vi "ProcessBufferUpdates.vi"(11 "MockFAILCSettings":T1={"ModbusRxDataFIFO"="ModbusSubnetARxDataFIFO", "ModbusTxDataFIFO"="ModbusSubnetATxDataFIFO", "BufferUpdateFIFO"="MockFAILC1Command", "Code17Memory"="MockFAILC1Code17", "Code18Memory"="MockFAILC1Code18", "Code65Memory"="MockFAILC1Code65", "Code72Memory"="MockFAILC1Code72", "Code74Memory"="MockFAILC1Code74", "Code75Memory"="MockFAILC1Code75", "Code76Memory"="MockFAILC1Code76", "Code80Memory"="MockFAILC1Code80", "Code110Memory"="MockFAILC1Code110", "Code120Memory"="MockFAILC1Code120", "Code121Memory"="MockFAILC1Code121", "CRCDataFIFO"="MockFAILC1CRCDataFIFO", "CRCCalculateFIFO"="MockFAILC1CRCCalculateFIFO", "CRCFIFO"="MockFAILC1CRCFIFO"}) -> ()   [LabVIEW 2016, in "FPGAMockFAILC.lvlib"]
uses:
  FPGAMockFAILC.lvlib
  DataTypes/MockFAILCSettings.ctl
  FPGAMockHPILC/DataTypes/MockHPBufferUpdateLoopData.ctl
  FPGAMockHPILC/DataTypes/MockHPBufferUpdateStates.ctl
  <vilib>/Platform/TimedLoop/XDataNode/timing_clust.ctl
  <vilib>/Platform/TimedLoop/XDataNode/nitl_modes.ctl
  <vilib>/Platform/TimedLoop/XDataNode/wakeup.ctl
  <vilib>/rvi/Emulation/niFpgaSctlEmulationGetInTimedLoop.vi
  <vilib>/rvi/Emulation/niFpgaEmulationReportErrorSimple.vi
  <vilib>/rvi/Emulation/niFpgaGetClockAttributes.vi
  <vilib>/rvi/Emulation/niFpgaCriticalErrorInLSC.vi
  <vilib>/rvi/DataTransferAndStorage/Container/Common/niFpgaContainerExecOnDevCompGetState.vi
  <vilib>/rvi/Emulation/niFpgaEmulationIsFPGAContextNoSignature.vi
  <vilib>/rvi/errors/niFpgaSetErrorForExecOnDevCompSimple.vi
  <vilib>/rvi/eio/common/nirviEmuReportErrorAndStop.vi
  <vilib>/rvi/DataTransferAndStorage/Container/Common/niFpgaContainerGetUniqueNameForEmu.vi
  <vilib>/rvi/FIFO/Fifo_Resource/nirvififoEmulationSetSize.vi
  <vilib>/rvi/FIFO/Fifo_Resource/nirviFifoEmulationQueueMgr.vi
  <instcachedir>/0/nirviFifoEmulationQueueMgr_E5CAEC123FF24DC58D834DCA3CDAA9B5.lvgen/nirviFifoEmulationQueueMgr_E5CAEC123FF24DC58D834DCA3CDAA9B5_009.vi
  <vilib>/rvi/FIFO/Fifo_Resource/nirvififoEmulationDetermineInputValidOut.vi
  <vilib>/rvi/FIFO/Fifo_Resource/nirvififoEmulationCreateLock.vi
  <vilib>/rvi/Emulation/niFpgaProcessEmulError.vi
  <vilib>/rvi/FIFO/Fifo_Resource/nirvififoEmulationObtainLock.vi
  <vilib>/rvi/FIFO/Fifo_Resource/nirvififoEmulationReleaseLock.vi
  <vilib>/rvi/occurrence/nirviWaitOnOccurrenceBase.vi
  <vilib>/rvi/errors/nirviReportUnexpectedCaseInternalError.vi
  <vilib>/rvi/errors/nirviReportUnexpectedCaseInternalError (U32).vi
  <vilib>/Utility/error.llb/Clear Errors.vi
  <vilib>/rvi/interface/RandomDataEmulation/niFpgaRandomDataHandleErrors.vi
  <vilib>/rvi/Memory/Memory_Emulation/niFpgaMemoryEmulationCacheClearOnFirstRun.vi
  <vilib>/rvi/Memory/Memory_Emulation/nirvimemoryEmulationManagerCache_MakeExclusive.vi
  <vilib>/rvi/Memory/Memory_Emulation/niFpgaMemoryEmulationValidateCache.vi
  <vilib>/rvi/Memory/Memory_Emulation/nirvimemoryEmulationManagerCache_InsertValue.vi
  <vilib>/rvi/Memory/Memory_Emulation/nirvimemoryEmulationManagerCache_ReleaseExclusive.vi
  <vilib>/rvi/Memory/Memory_Emulation/nirvimemoryEmulationManagerCache_GetValue.vi
  <vilib>/rvi/Memory/Memory_Emulation/nirvimemoryEmulationManagerCache_SetValue.vi
  <vilib>/rvi/Emulation/niFpgaSctlEmulationResourceMgr.vi
  <vilib>/Platform/TimedLoop/XDataNode/XDataNode.xnode
  <vilib>/rvi/DataTransferAndStorage/Container/XNode/niFpgaContainer.xnode
  <vilib>/rvi/FIFO/Fifo_Resource/niFpgaFifoEmulationRefIn.vi
  <vilib>/rvi/Memory/Memory_Emulation/niFpgaMemoryEmulationRefIn.vi
  <vilib>/Platform/TimedLoop/XDataNode/XDNodeRunTimeDep.lvlib
  FPGAMockHPILC/FPGAMockHPILC.lvlib
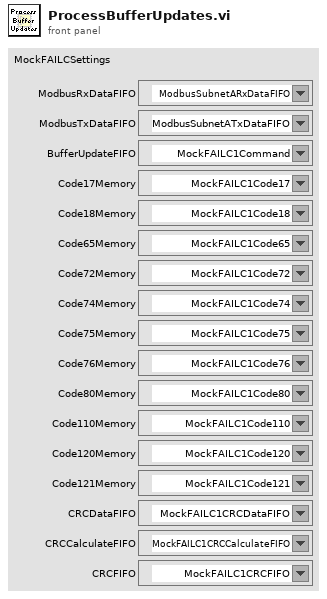
[diagram p1: front panel]
types:
  T1 = typedef "FPGAMockFAILC.lvlib/MockFAILCSettings.ctl" = cluster{"ModbusRxDataFIFO":refnum<k21>, "ModbusTxDataFIFO":refnum<k21>, "BufferUpdateFIFO":refnum<k21>, "Code17Memory":refnum<k21>, "Code18Memory":refnum<k21>, "Code65Memory":refnum<k21>, "Code72Memory":refnum<k21>, "Code74Memory":refnum<k21>, "Code75Memory":refnum<k21>, "Code76Memory":refnum<k21>, "Code80Memory":refnum<k21>, "Code110Memory":refnum<k21>, "Code120Memory":refnum<k21>, "Code121Memory":refnum<k21>, "CRCDataFIFO":refnum<k21>, "CRCCalculateFIFO":refnum<k21>, "CRCFIFO":refnum<k21>}
  T2 = typedef "FPGAMockHPILC.lvlib/MockHPBufferUpdateLoopData.ctl" = cluster{"BufferUpdateLoopStates":T3, "Address":u32, "Function":u8, "Length":u32, "Data":u8, "Index":u32}
  T3 = typedef "FPGAMockHPILC.lvlib/MockHPBufferUpdateStates.ctl" = enum16{"ReadAddress", "ReadFunction", "ReadLength", "ReadData", "WriteData"}
  T4 = typedef "XDNodeRunTimeDep.lvlib/timing_clust.ctl" = cluster{"Expected End [f-1]":u64, "Actual End [f-1]":u64, "Finished Late? [f-1]":bool, "Expected End [i-1]":u64, "Actual End [i-1]":u64, "Finished Late? [i-1]":bool, "Expected Start [i]":u64, "Actual Start [i]":u64, "Expected Start [f]":u64, "Actual Start [f]":u64, "Source Name":string, "Structure Name":string, "Period":i64, "Deadline":i64, "Offset":i64, "Start":i64, "Priority":i32, "Timeout":i32, "Mode":T5, "Wakeup Reason":T6, "Error":errorcluster, "Source Type":string, "Secondary Source Type":string, "Global End Time":u64, "Global Start Time":u64, "Frame Duration":u64, "Iteration Duration":u64, "Assigned CPU":i32, "I/O Scan Engine Mode":u32}
  T5 = typedef "XDNodeRunTimeDep.lvlib/nitl_modes.ctl" = enum32{"No Change", "Process missed periods, maintain original phase", "Discard missed periods, maintain original phase", "Process missed periods, ignore original phase", "Discard missed periods, ignore original phase"}
  T6 = typedef "XDNodeRunTimeDep.lvlib/wakeup.ctl" = enum32{"Normal", "Aborted", "Asynchronous wakeup", "Timing source error", "Timed loop error", "Timeout"}
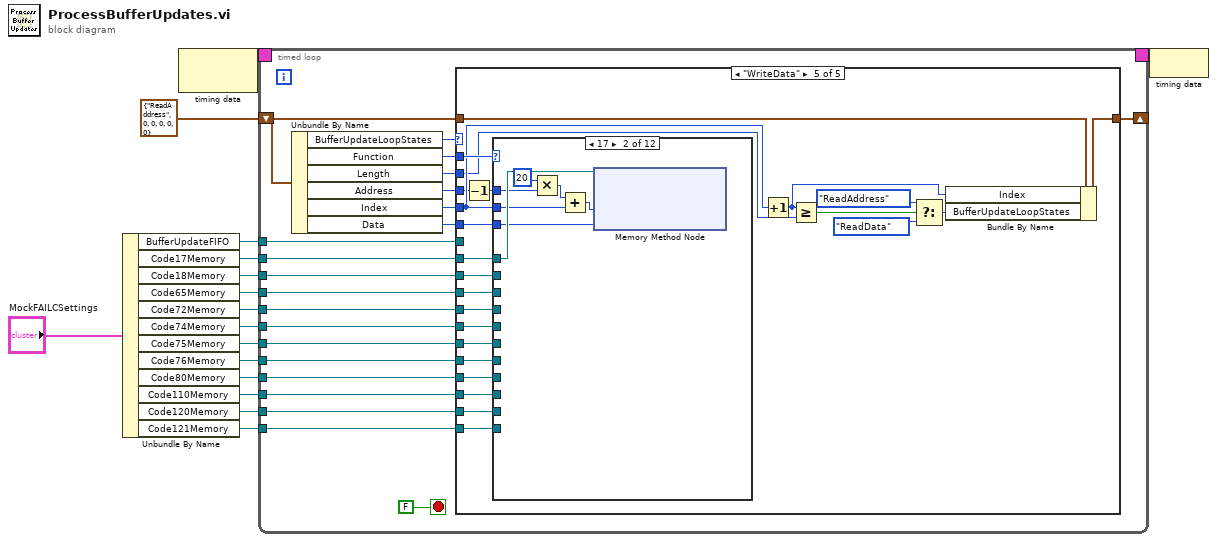
[diagram p0: block diagram]
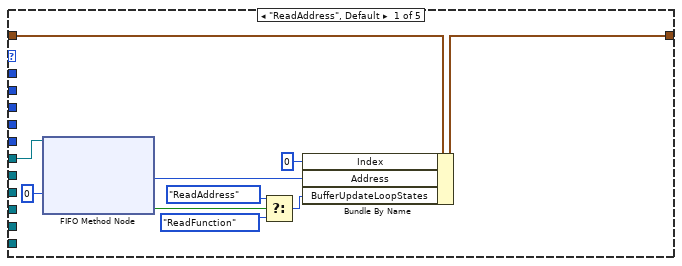
[diagram p2: hidden frame]
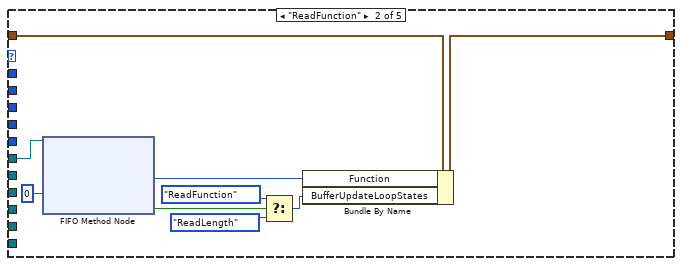
[diagram p3: hidden frame]
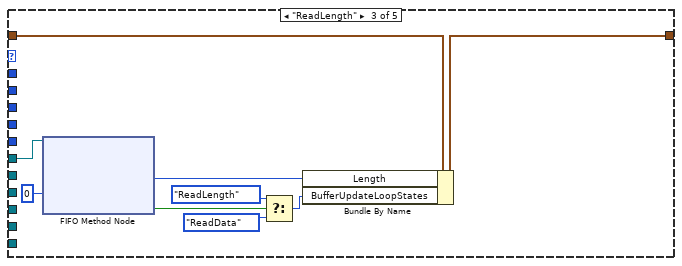
[diagram p4: hidden frame]
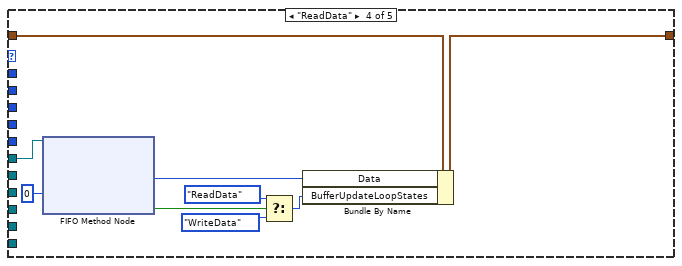
[diagram p5: hidden frame]
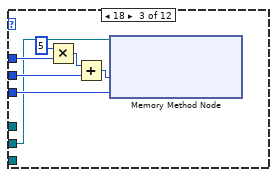
[diagram p7: hidden frame]
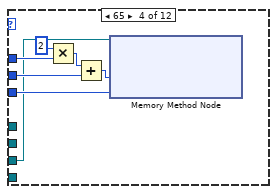
[diagram p8: hidden frame]
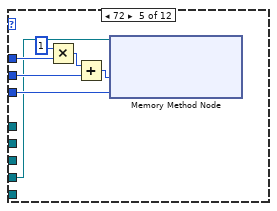
[diagram p9: hidden frame]
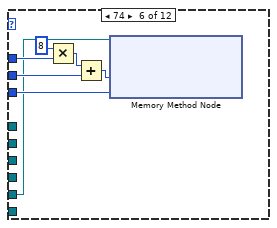
[diagram p10: hidden frame]
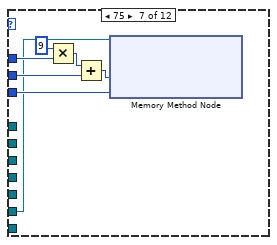
[diagram p11: hidden frame]
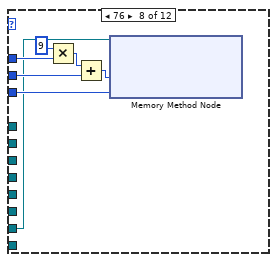
[diagram p12: hidden frame]
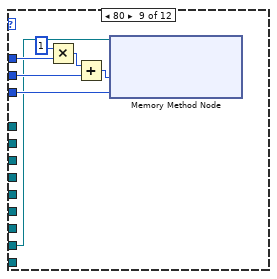
[diagram p13: hidden frame]
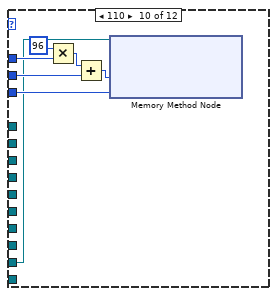
[diagram p14: hidden frame]
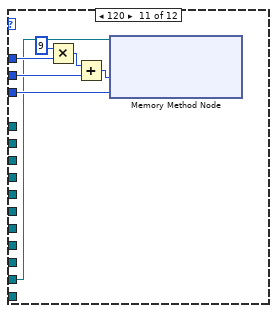
[diagram p15: hidden frame]
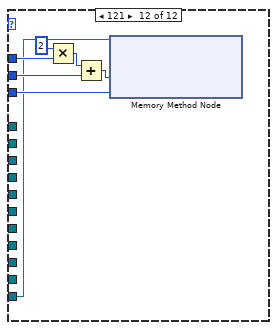
[diagram p16: hidden frame]
diagram:
  n1 = Unbundle By Name("MockFAILCSettings") -> ("BufferUpdateFIFO"=w13:refnum<k21>, "Code17Memory"=w12:refnum<k21>, "Code18Memory"=w11:refnum<k21>, "Code65Memory"=w10:refnum<k21>, "Code72Memory"=w9:refnum<k21>, "Code74Memory"=w8:refnum<k21>, "Code75Memory"=w7:refnum<k21>, "Code76Memory"=w6:refnum<k21>, "Code80Memory"=w5:refnum<k21>, "Code110Memory"=w3:refnum<k21>, "Code120Memory"=w2:refnum<k21>, "Code121Memory"=w1:refnum<k21>)
  n2 = node-c288() -> (w16:T4)  [unwired: 1 in]
  n3 = timed-loop {
    timing: w16 -> [_]
    timing-out: [_] -> w15
    tunnel: w13 -> [w36]
    tunnel: w12 -> [w28]
    tunnel: w11 -> [w27]
    tunnel: w10 -> [w26]
    tunnel: w9 -> [w25]
    tunnel: w8 -> [w24]
    tunnel: w7 -> [w23]
    tunnel: w6 -> [w22]
    tunnel: w5 -> [w21]
    shift-right: [w30] -> _
    shift-left: T2 {"BufferUpdateLoopStates"=enum."ReadAddress", "Address"=0, "Function"=0, "Length"=0, "Data"=0, "Index"=0} ("MockHPBufferUpdateLoopData") -> [w35]
    tunnel: w3 -> [w19]
    tunnel: w2 -> [w18]
    tunnel: w1 -> [w17]
    stop <- FALSE stop-if-true
    n4 = Unbundle By Name(w35) -> ("BufferUpdateLoopStates"=w37:T3, "Function"=w34:u8, "Length"=w33:u32, "Address"=w32:u32, "Index"=w31:u32, "Data"=w29:u8)
    n5 = case shown="\"WriteData\"" w37 {
      tunnel: w36 -> [w47 w56 w65 w74 _]
      tunnel: w35 -> [w40 w49 w58 w67 w96]
      tunnel: w34 -> [_ _ _ _ w94]
      tunnel: w33 -> [_ _ _ _ w90]
      tunnel: w32 -> [_ _ _ _ w79]
      tunnel: w31 -> [_ _ _ _ w91]
      tunnel: [w39 w48 w57 w66 w95] -> w30
      tunnel: w29 -> [_ _ _ _ w92]
      tunnel: w28 -> [_ _ _ _ w93]
      tunnel: w27 -> [_ _ _ _ w86]
      tunnel: w26 -> [_ _ _ _ w85]
      tunnel: w25 -> [_ _ _ _ w84]
      tunnel: w24 -> [_ _ _ _ w83]
      tunnel: w23 -> [_ _ _ _ w82]
      tunnel: w22 -> [_ _ _ _ w81]
      tunnel: w21 -> [_ _ _ _ w80]
      tunnel: w19 -> [_ _ _ _ w77]
      tunnel: w18 -> [_ _ _ _ w76]
      tunnel: w17 -> [_ _ _ _ w75]
      frame "ReadAddress", Default {
        n6 = xnode ("FIFO Method Node")("Timeout"=0, "FIFO In"=w47) -> ("Element"=w42:u8, "Timed Out?"=w46:bool)  [unwired: 1 out]
        n7 = Select(t=MockHPBufferUpdateStates."ReadAddress" ("f"), s=w46, f=MockHPBufferUpdateStates."ReadFunction") -> (s? t:f=w41:T3)
        n8 = Bundle By Name(cluster=w40, "Index"=u8 0, "Address"=w42, "BufferUpdateLoopStates"=w41) -> (w39:T2)
      }
      frame "ReadFunction" {
        n9 = xnode ("FIFO Method Node")("Timeout"=0, "FIFO In"=w56) -> ("Element"=w51:u8, "Timed Out?"=w55:bool)  [unwired: 1 out]
        n10 = Select(t=MockHPBufferUpdateStates."ReadFunction" ("f"), s=w55, f=MockHPBufferUpdateStates."ReadLength") -> (s? t:f=w50:T3)
        n11 = Bundle By Name(cluster=w49, "Function"=w51, "BufferUpdateLoopStates"=w50) -> (w48:T2)
      }
      frame "ReadLength" {
        n12 = xnode ("FIFO Method Node")("Timeout"=0, "FIFO In"=w65) -> ("Element"=w60:u8, "Timed Out?"=w64:bool)  [unwired: 1 out]
        n13 = Select(t=MockHPBufferUpdateStates."ReadLength" ("f"), s=w64, f=MockHPBufferUpdateStates."ReadData") -> (s? t:f=w59:T3)
        n14 = Bundle By Name(cluster=w58, "Length"=w60, "BufferUpdateLoopStates"=w59) -> (w57:T2)
      }
      frame "ReadData" {
        n15 = xnode ("FIFO Method Node")("Timeout"=0, "FIFO In"=w74) -> ("Element"=w69:u8, "Timed Out?"=w73:bool)  [unwired: 1 out]
        n16 = Select(t=MockHPBufferUpdateStates."ReadData" ("f"), s=w73, f=MockHPBufferUpdateStates."WriteData") -> (s? t:f=w68:T3)
        n17 = Bundle By Name(cluster=w67, "Data"=w69, "BufferUpdateLoopStates"=w68) -> (w66:T2)
      }
      frame "WriteData" {
        n18 = Decrement(x=w79) -> (x-1=w78:u32)
        n19 = case shown="17" w94 {
          tunnel: w93 -> [_ w105 _ _ _ _ _ _ _ _ _ _]
          tunnel: w92 -> [_ w104 w112 w119 w126 w133 w140 w147 w154 w161 w168 w175]
          tunnel: w91 -> [_ w102 w110 w117 w124 w131 w138 w145 w152 w159 w166 w173]
          tunnel: w78 -> [_ w100 w108 w115 w122 w129 w136 w143 w150 w157 w164 w171]
          tunnel: w86 -> [_ _ w106 _ _ _ _ _ _ _ _ _]
          tunnel: w85 -> [_ _ _ w113 _ _ _ _ _ _ _ _]
          tunnel: w84 -> [_ _ _ _ w120 _ _ _ _ _ _ _]
          tunnel: w83 -> [_ _ _ _ _ w127 _ _ _ _ _ _]
          tunnel: w82 -> [_ _ _ _ _ _ w134 _ _ _ _ _]
          tunnel: w81 -> [_ _ _ _ _ _ _ w141 _ _ _ _]
          tunnel: w80 -> [_ _ _ _ _ _ _ _ w148 _ _ _]
          tunnel: w77 -> [_ _ _ _ _ _ _ _ _ w155 _ _]
          tunnel: w76 -> [_ _ _ _ _ _ _ _ _ _ w162 _]
          tunnel: w75 -> [_ _ _ _ _ _ _ _ _ _ _ w169]
          frame 0, Default {
          }
          frame 17 {
            n20 = Multiply(x=u32 20, y=w100) -> (x*y=w103:u32)
            n21 = Add(x=w103, y=w102) -> (x+y=w101:u32)
            n22 = xnode ("Memory Method Node")("Address"=w101, "Data"=w104, "Memory In"=w105) -> ()  [unwired: 1 out]
          }
          frame 18 {
            n23 = Multiply(x=u32 5, y=w108) -> (x*y=w111:u32)
            n24 = Add(x=w111, y=w110) -> (x+y=w109:u32)
            n25 = xnode ("Memory Method Node")("Address"=w109, "Data"=w112, "Memory In"=w106) -> ()  [unwired: 1 out]
          }
          frame 65 {
            n26 = Multiply(x=u32 2, y=w115) -> (x*y=w118:u32)
            n27 = Add(x=w118, y=w117) -> (x+y=w116:u32)
            n28 = xnode ("Memory Method Node")("Address"=w116, "Data"=w119, "Memory In"=w113) -> ()  [unwired: 1 out]
          }
          frame 72 {
            n29 = Multiply(x=u32 1, y=w122) -> (x*y=w125:u32)
            n30 = Add(x=w125, y=w124) -> (x+y=w123:u32)
            n31 = xnode ("Memory Method Node")("Address"=w123, "Data"=w126, "Memory In"=w120) -> ()  [unwired: 1 out]
          }
          frame 74 {
            n32 = Multiply(x=u32 8, y=w129) -> (x*y=w132:u32)
            n33 = Add(x=w132, y=w131) -> (x+y=w130:u32)
            n34 = xnode ("Memory Method Node")("Address"=w130, "Data"=w133, "Memory In"=w127) -> ()  [unwired: 1 out]
          }
          frame 75 {
            n35 = Multiply(x=u32 9, y=w136) -> (x*y=w139:u32)
            n36 = Add(x=w139, y=w138) -> (x+y=w137:u32)
            n37 = xnode ("Memory Method Node")("Address"=w137, "Data"=w140, "Memory In"=w134) -> ()  [unwired: 1 out]
          }
          frame 76 {
            n38 = Multiply(x=u32 9, y=w143) -> (x*y=w146:u32)
            n39 = Add(x=w146, y=w145) -> (x+y=w144:u32)
            n40 = xnode ("Memory Method Node")("Address"=w144, "Data"=w147, "Memory In"=w141) -> ()  [unwired: 1 out]
          }
          frame 80 {
            n41 = Multiply(x=u32 1, y=w150) -> (x*y=w153:u32)
            n42 = Add(x=w153, y=w152) -> (x+y=w151:u32)
            n43 = xnode ("Memory Method Node")("Address"=w151, "Data"=w154, "Memory In"=w148) -> ()  [unwired: 1 out]
          }
          frame 110 {
            n44 = Multiply(x=u32 96, y=w157) -> (x*y=w160:u32)
            n45 = Add(x=w160, y=w159) -> (x+y=w158:u32)
            n46 = xnode ("Memory Method Node")("Address"=w158, "Data"=w161, "Memory In"=w155) -> ()  [unwired: 1 out]
          }
          frame 120 {
            n47 = Multiply(x=u32 9, y=w164) -> (x*y=w167:u32)
            n48 = Add(x=w167, y=w166) -> (x+y=w165:u32)
            n49 = xnode ("Memory Method Node")("Address"=w165, "Data"=w168, "Memory In"=w162) -> ()  [unwired: 1 out]
          }
          frame 121 {
            n50 = Multiply(x=u32 2, y=w171) -> (x*y=w174:u32)
            n51 = Add(x=w174, y=w173) -> (x+y=w172:u32)
            n52 = xnode ("Memory Method Node")("Address"=w172, "Data"=w175, "Memory In"=w169) -> ()  [unwired: 1 out]
          }
        }
        n53 = Increment(x=w91) -> (x+1=w87:u32)
        n54 = Greater Or Equal?(x=w87, y=w90) -> (x >= y?=w89:bool)
        n55 = Select(t=MockHPBufferUpdateStates."ReadAddress" ("f"), s=w89, f=MockHPBufferUpdateStates."ReadData") -> (s? t:f=w88:T3)
        n56 = Bundle By Name(cluster=w96, "Index"=w87, "BufferUpdateLoopStates"=w88) -> (w95:T2)
      }
    }
  }
  n57 = node-c288(w15) -> ()
